vi "Write Duration.vi"(8 "error in (no error)":errorcluster, 10 "Duration":dbl, 11 "Write Duration Msg in":refnum<class "Write Duration Msg.lvclass">) -> (0 "error out":errorcluster, 3 "Write Duration Msg out":refnum<class "Write Duration Msg.lvclass">)   [LabVIEW 2015, in "Write Duration Msg.lvclass"]
uses:
  Write Duration Msg.lvclass
  Write Duration Msg.lvclass/Write Duration Msg.ctl
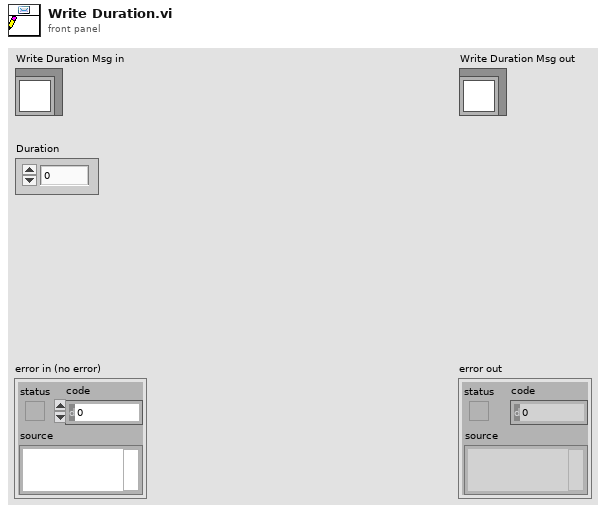
[diagram p1: front panel]
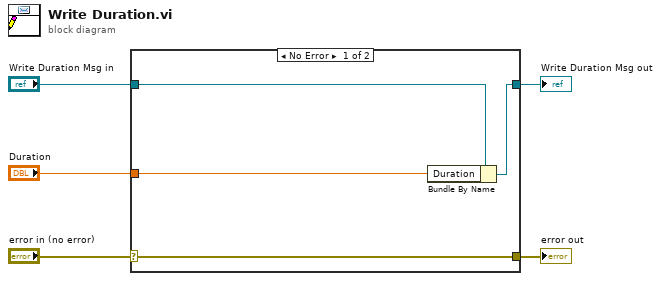
[diagram p0: block diagram]
diagram:
  n1 = case shown="No Error" "error in (no error)" {
    selector: "error in (no error)" -> [w9 w10]
    tunnel: [w9 w10] -> w4
    tunnel: [w7 w11] -> w2
    tunnel: "Write Duration Msg in" -> [w8 w11]
    tunnel: "Duration" -> [w6 _]
    frame No Error {
      n2 = Bundle By Name(cluster=w8, "Duration"=w6) -> (w7:refnum<class "Write Duration Msg.lvclass">)
    }
    frame Error {
    }
  }
  "error out" <- w4
  "Write Duration Msg out" <- w2
